vi "UsrProfiles-User login.vi"(8 "error in (no error)":errorcluster, 11 "Access source (Soft init)":T1(ring)) -> (0 "error out":errorcluster)   [LabVIEW 2017]
uses:
  Typedefs/Set Main VI cursor.ctl
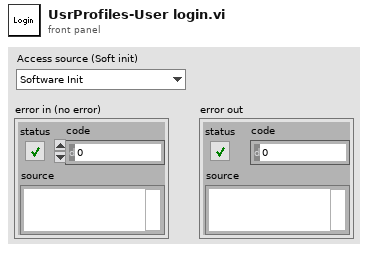
[diagram p1: front panel]
types:
  T1 = enum16{"Software Init", "User menu", "Switch User button"}
  T2 = typedef "Set Main VI cursor.ctl" = enum16{"Release busy cursor", "Set busy cursor"}
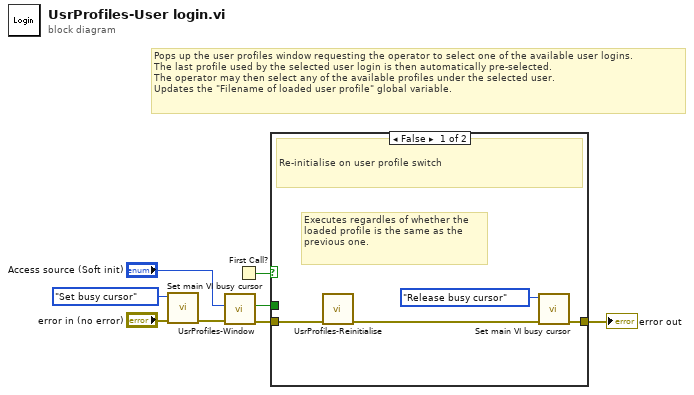
[diagram p0: block diagram]
diagram:
  # "Pops up the user profiles window requesting the operator to select one of the available user logins.\nThe last profile used by the selected user login is then automatically pre-selected.\nThe operator may then select any of the available profiles under the selected user.\nUpdates the \"Filename of loaded user profile\" global variable."
  n1 = call "Set main VI busy cursor.vi"("error in (no error)"="error in (no error)", "Main VI's cursor"=Set_Main_VI_cursor."Set busy cursor") -> ("error out"=w6:errorcluster)  [unwired: 9 in]
  n2 = call "UsrProfiles-Window.vi"("error in (no error)"=w6, "Access source"="Access source (Soft init)") -> ("error out"=w2:errorcluster, "Profile change"=w1:bool)  [unwired: 8 in]
  n3 = First Call?() -> (First Call?: T/F=w3:bool)
  n4 = case shown="False" w3 {
    tunnel: w2 -> [w12 w13]
    tunnel: [w9 w13] -> w8
    tunnel: w1 -> [_ _]
    frame False {
      # "Executes regardles of whether the loaded profile is the same as the previous one."
      # "Re-initialise on user profile switch"
      n5 = call "UsrProfiles-Reinitialise.vi"("error in"=w12) -> ("error out"=w10:errorcluster)  [unwired: 10 in]
      n6 = call "Set main VI busy cursor.vi"("error in (no error)"=w10, "Main VI's cursor"=Set_Main_VI_cursor."Release busy cursor") -> ("error out"=w9:errorcluster)  [unwired: 9 in]
    }
    frame True {
      # "Main screen busy cursor is reset further \ndown the software initialisation sequence."
      # "Software initialisation"
    }
  }
  "error out" <- w8
